vi "scroll.vi"(8 "error in (no error)":errorcluster, 9 "axis info":T1, 10 "keys pressed":T2(array[ring]), 11 "ScanHeadMH100729FPGA in":refnum<class "ScanHeadMH100729FPGA.lvclass">) -> (0 "error out":errorcluster, 3 "ScanHeadMH100729FPGA out":refnum<class "ScanHeadMH100729FPGA.lvclass">)   [LabVIEW 2010, in "ScanHeadMH100729FPGA.lvclass"]
uses:
  ScanHeadMH100729FPGA.lvclass
  ScanHeadMH100729FPGA.lvclass/ScanHeadMH100729FPGA.ctl
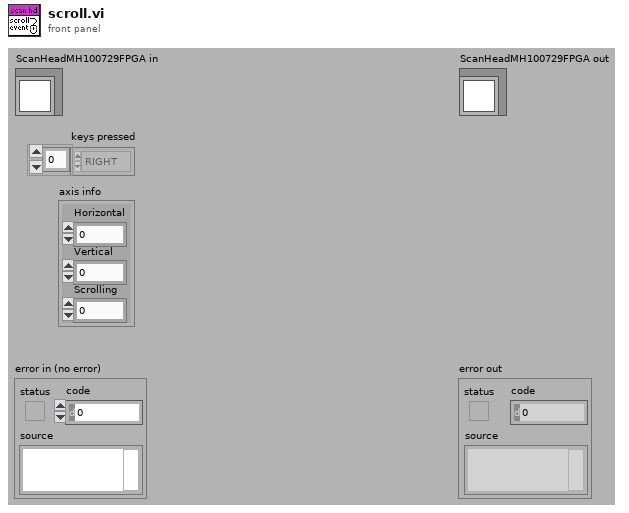
[diagram p1: front panel]
types:
  T1 = cluster{"Horizontal":i32, "Vertical":i32, "Scrolling":i32}
  T2 = enum16{"0", "1", "2", "3", "4", "5", "6", "7", "8", "9", "A", "B", "C", "D", "E", "F", "G", "H", "I", "J", "K", "L", "M", "N", "O", "P", "Q", "R", "S", "T", "U", "V", "W", "X", "Y", "Z", "F1", "F2", "F3", "F4", "F5", "F6", "F7", "F8", "F9", "F10", "F11", "F12", "F13", "F14", "F15", "ADD", "BACK", "BACKSLASH", "CAPITAL", "COMMA", "DECIMAL", "DELETE", "DIVIDE", "DOWN", "END", "EQUALS", "ESCAPE", "GRAVE (`)", "HOME", "INSERT", "LBRACKET", "LCONTROL", "LEFT", "L ALT", "LSHIFT", "LWIN", "MINUS", "MULTIPLY", "NEXT", "NUMLOCK", "NUMPAD_0", "NUMPAD_1", "NUMPAD_2", "NUMPAD_3", "NUMPAD_4", "NUMPAD_5", "NUMPAD_6", "NUMPAD_7", "NUMPAD_8", "NUMPAD_9", "PAUSE", "PERIOD", "PRIOR (PG UP)", "RBRACKET", "RCONTROL", "RETURN", "RIGHT", "R ALT", "RSHIFT", "RWIN", "SCROLL", "SEMICOLON", "SLASH", "SPACE", "SUBTRACT", "TAB", "UP", "ENTER (num pad)", "' (quote)"}[]
  T3 = enum16{"0", "1", "2", "3", "4", "5", "6", "7", "8", "9", "A", "B", "C", "D", "E", "F", "G", "H", "I", "J", "K", "L", "M", "N", "O", "P", "Q", "R", "S", "T", "U", "V", "W", "X", "Y", "Z", "F1", "F2", "F3", "F4", "F5", "F6", "F7", "F8", "F9", "F10", "F11", "F12", "F13", "F14", "F15", "ADD", "BACK", "BACKSLASH", "CAPITAL", "COMMA", "DECIMAL", "DELETE", "DIVIDE", "DOWN", "END", "EQUALS", "ESCAPE", "GRAVE (`)", "HOME", "INSERT", "LBRACKET", "LCONTROL", "LEFT", "L ALT", "LSHIFT", "LWIN", "MINUS", "MULTIPLY", "NEXT", "NUMLOCK", "NUMPAD_0", "NUMPAD_1", "NUMPAD_2", "NUMPAD_3", "NUMPAD_4", "NUMPAD_5", "NUMPAD_6", "NUMPAD_7", "NUMPAD_8", "NUMPAD_9", "PAUSE", "PERIOD", "PRIOR (PG UP)", "RBRACKET", "RCONTROL", "RETURN", "RIGHT", "R ALT", "RSHIFT", "RWIN", "SCROLL", "SEMICOLON", "SLASH", "SPACE", "SUBTRACT", "TAB", "UP", "ENTER (num pad)", "' (quote)"}
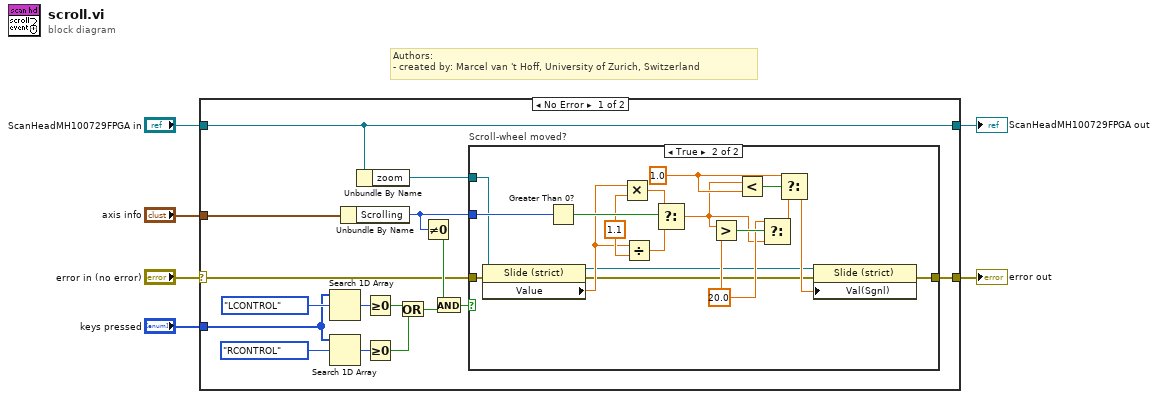
[diagram p0: block diagram]
diagram:
  # "Authors: \n- created by: Marcel van 't Hoff, University of Zurich, Switzerland"
  n1 = case shown="No Error" "error in (no error)" {
    selector: "error in (no error)" -> [w10 w43]
    tunnel: [w9 w43] -> w5
    tunnel: [w8 w42] -> w3
    tunnel: "ScanHeadMH100729FPGA in" -> [w8 w42]
    tunnel: "keys pressed" -> [w20 _]
    tunnel: "axis info" -> [w22 _]
    frame No Error {
      n2 = Search 1D Array(1D array=w20, element=T3."LCONTROL") -> (index of element=w16:i32)  [unwired: 1 in]
      n3 = Search 1D Array(1D array=w20, element=T3."RCONTROL") -> (index of element=w18:i32)  [unwired: 1 in]
      n4 = Unbundle By Name(w22) -> ("Scrolling"=w11:i32)
      n5 = Unbundle By Name(w8) -> ("zoom"=w7:refnum<vi>)
      n6 = Greater Or Equal To 0?(x=w16) -> (x >= 0?=w15:bool)
      n7 = Greater Or Equal To 0?(x=w18) -> (x >= 0?=w17:bool)
      n8 = Or(x=w15, y=w17) -> (x .or. y?=w14:bool)
      n9 = Not Equal To 0?(x=w11) -> (x != 0?=w13:bool)
      n10 = And(x=w13, y=w14) -> (x .and. y?=w12:bool)
      n11 = case "Scroll-wheel moved?" shown="True" w12 {
        tunnel: [w23 w30] -> w9
        tunnel: w10 -> [w23 w27]
        tunnel: w11 -> [_ w31]
        tunnel: w7 -> [_ w25]
        frame False {
        }
        frame True {
          w34 = 20.0 ("y")
          w36 = 1.0 ("y")
          w38 = 1.1 ("y")
          n12 = property class="Slide (strict)"(reference=w25, error in=w27) -> (reference out=w24:refnum<vi>, error out=w26:errorcluster, "Value"=w28:dbl)
          n13 = Greater Than 0?(x=w31) -> (x > 0?=w41:bool)
          n14 = Multiply(x=w28, y=w38) -> (x*y=w40:dbl)
          n15 = Divide(x=w28, y=w38) -> (x/y=w39:dbl)
          n16 = Select(t=w40, s=w41, f=w39) -> (s? t:f=w32:dbl)
          n17 = Greater?(x=w32, y=w34) -> (0:w35:bool)
          n18 = Less?(x=w32, y=w36) -> (x < y?=w37:bool)
          n19 = Select(t=w34, s=w35, f=w32) -> (s? t:f=w33:dbl)
          n20 = Select(t=w36, s=w37, f=w33) -> (s? t:f=w29:dbl)
          n21 = property class="Slide (strict)"(reference=w24, error in=w26, "Val(Sgnl)"=w29) -> (error out=w30:errorcluster)  [unwired: 1 out]
        }
      }
    }
    frame Error {
    }
  }
  "error out" <- w5
  "ScanHeadMH100729FPGA out" <- w3
